vi "Test First Enqueued Return Value is Returned when Recording Expectation.vi"(8 "error in (no error)":errorcluster, 11 "Test Case In":refnum<class "Return Value Test.lvclass">) -> (0 "error out":errorcluster, 3 "Test Case Out":refnum<class "Return Value Test.lvclass">)   [LabVIEW 2020, in "Return Value Test.lvclass"]
uses:
  Return Value Test.lvclass
  4993e8ee-a06a-463a-9684-69129f64d5ce.vi
  Test Doubles/Test Interface Responsive Mock/Test Interface Responsive Mock.lvclass
  source/Expectations/One/One.lvclass
  <vilib>/Astemes/LUnit/Test Case.lvclass
  C:/git/astemes-lmock/source/Framework/Mock/Mock.lvclass
  C:/git/astemes-lmock/tests/Test Doubles/Test Interface Responsive Mock/Test Interface Responsive Mock.lvclass
  C:/git/astemes-lmock/tests/Test Doubles/Test Interface/Test Interface.lvclass
  C:/Program Files (x86)/National Instruments/LabVIEW 2020/vi.lib/Astemes/LUnit/Test Case.lvclass
  C:/Program Files (x86)/National Instruments/LabVIEW 2020/vi.lib/Astemes/LUnit/LUnit Runnable.lvclass
  C:/git/astemes-lmock/tests/Return Value Test/Return Value Test.lvclass
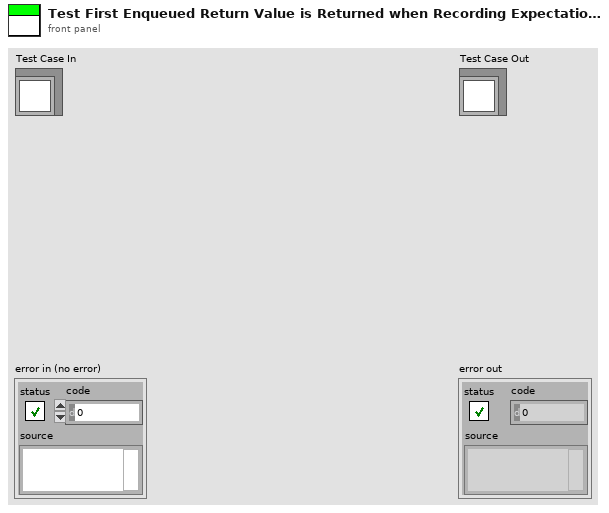
[diagram p1: front panel]
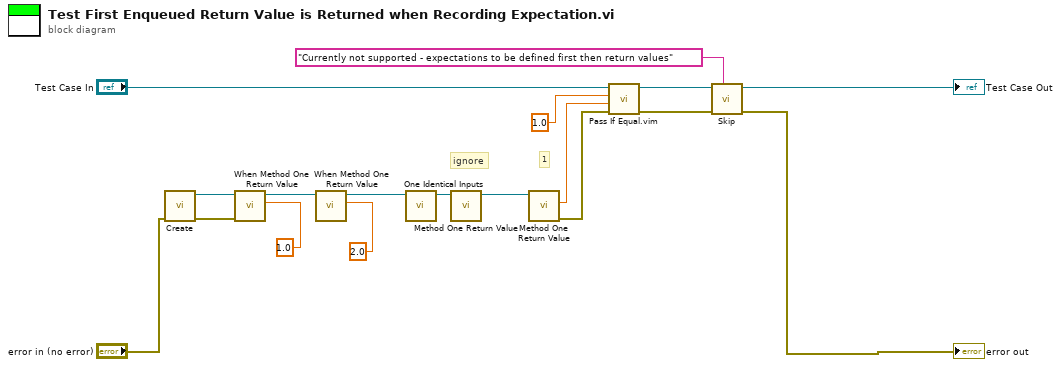
[diagram p0: block diagram]
diagram:
  # "ignore"
  # "1"
  n1 = call "Create.vi"("error in (no error)"="error in (no error)") -> ("error out"=w15:errorcluster, "Test Interface Mock Out"=w16:refnum<class "Test Interface Responsive Mock.lvclass">)  [unwired: 9 in]
  n2 = call "When Method One Return Value.vi"("Return Value"=1.0, "error in (no error)"=w15, "Test Interface Mock In"=w16) -> ("Test Interface Mock Out"=w14:refnum<class "Test Interface Responsive Mock.lvclass">)  [unwired: 8 in]
  n3 = call "When Method One Return Value.vi"("Return Value"=2.0, "Test Interface Mock In"=w14) -> ("Test Interface Mock Out"=w11:refnum<class "Test Interface Responsive Mock.lvclass">)  [unwired: 9 in]
  n4 = call "One Identical Inputs.vi"("Mock in"=w11) -> ("Mock out"=w6:refnum<class "Test Interface Responsive Mock.lvclass">)  [unwired: 9 in, 1 out]
  n5 = call-dynamic "Method One Return Value.vi"("Test Interface Mock in"=w6) -> ("Test Interface Mock out"=w5:refnum<class "Test Interface Responsive Mock.lvclass">)  [unwired: 8 in, 2 out]
  n6 = call-dynamic "Method One Return Value.vi"("Test Interface Mock in"=w5) -> ("error out"=w13:errorcluster, "Return Value"=w7:dbl)  [unwired: 8 in, 1 out]
  n7 = call "Pass If Equal.vim"("error in (no error)"=w13, "Actual"=w7, "Expected"=1.0 ("Return Value"), "LUnit Test Case In"="Test Case In") -> ("error out"=w17:errorcluster, "LUnit Test Case Out"=w3:refnum<class "Return Value Test.lvclass">)  [unwired: 6 in]
  n8 = call <vilib>:"Skip.vi"("Description"="Currently not supported - expectations to be defined first then return values", "error in (no error)"=w17, "LUnit Test Case In"=w3) -> ("error out"=→"error out":errorcluster, "LUnit Test Case Out"=→"Test Case Out":refnum<class "Return Value Test.lvclass">)  [unwired: 7 in]
